vi "SDCCB Send Command.vi"(0 "VISA Ref":refnum<visa-resource-name>, 2 "Wait for Reply (T)":bool=TRUE, 7 "Command":string, 11 "Error In":errorcluster) -> (4 "VISA Ref Dup":refnum<visa-resource-name>, 8 "Reply":string, 15 "Error Out":errorcluster)   [LabVIEW 2020]
uses:
  <vilib>/Utility/error.llb/whitespace.ctl
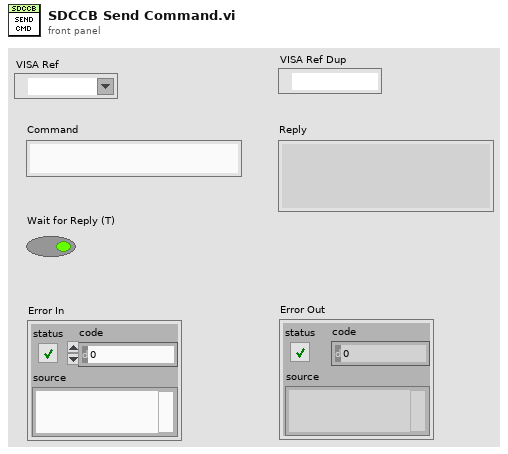
[diagram p1: front panel]
types:
  T1 = typedef "whitespace.ctl" = u16
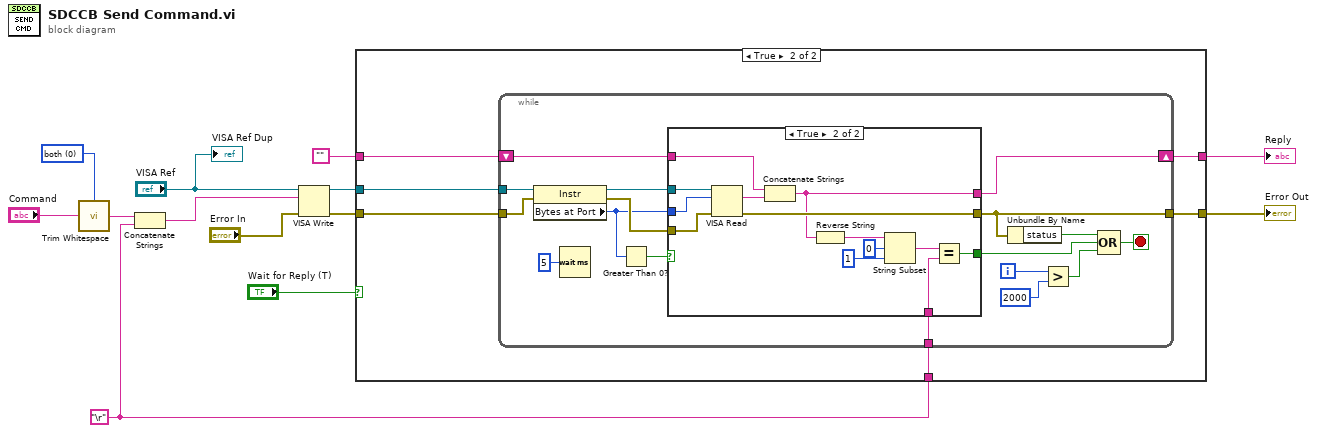
[diagram p0: block diagram]
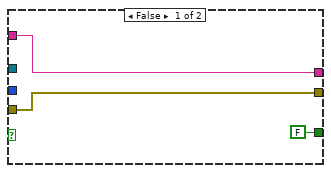
[diagram p3: hidden frame]
diagram:
  w1 = "\r"
  w12 = T1 0 items=["both", "start of string", "end of string"] ("location (both)")
  n1 = call <vilib>:"Trim Whitespace.vi"("string"="Command", "location (both)"=w12) -> ("trimmed string"=w11:string)
  n2 = Concatenate Strings(w11, w1) -> (w10:string)
  n3 = VISA Write(VISA resource name="VISA Ref", write buffer=w10, error in (no error)="Error In") -> (VISA resource name out=w9:refnum<visa-resource-name>, error out=w8:errorcluster)  [unwired: 1 out]
  n4 = case shown="True" "Wait for Reply (T)" {
    tunnel: w9 -> [_ w18]
    tunnel: w8 -> [w15 w17]
    tunnel: "" -> [w14 w21]
    tunnel: [w14 w20] -> w2
    tunnel: [w15 w19] -> w4
    tunnel: w1 -> [_ w16]
    frame False {
    }
    frame True {
      n5 = while {
        tunnel: w18 -> [w38]
        tunnel: w17 -> [w37]
        shift-right: [w26] -> w20
        shift-left: w21 -> [w27]
        tunnel: [w23] -> w19
        tunnel: w16 -> [w22]
        i -> [w36]
        stop <- w33 stop-if-true
        n6 = property class="Instr"(reference=w38, error in=w37) -> (reference out=w29:refnum<visa-resource-name>, error out=w30:errorcluster, "Bytes at Port"=w28:u32)
        n7 = Wait (ms)(milliseconds to wait=u32 5) -> ()  [unwired: 1 out]
        n8 = Greater Than 0?(x=w28) -> (x > 0?=w31:bool)
        n9 = case shown="True" w31 {
          tunnel: w30 -> [w40 w53]
          tunnel: w29 -> [_ w54]
          tunnel: w28 -> [_ w52]
          tunnel: w27 -> [w41 w51]
          tunnel: [w41 w48] -> w26
          tunnel: [w40 w49] -> w23
          tunnel: [FALSE w43] -> w24
          tunnel: w22 -> [_ w42]
          frame False {
          }
          frame True {
            n10 = VISA Read(VISA resource name=w54, byte count=w52, error in (no error)=w53) -> (read buffer=w50:string, error out=w49:errorcluster)  [unwired: 2 out]
            n11 = Concatenate Strings(w51, w50) -> (w48:string)
            n12 = Reverse String(1:w48) -> (0:w47:string)
            n13 = String Subset(string=w47, offset (0)=0, length (rest)=1 ("length (rest)")) -> (substring=w44:string)
            n14 = Equal?(x=w44, y=w42) -> (x = y?=w43:bool)
          }
        }
        n15 = Unbundle By Name(w23) -> ("status"=w25:bool)
        n16 = Greater?(x=w36, y=2000) -> (0:w34:bool)
        n17 = Compound Arithmetic op=OR(w25, w24, w34) -> (w33:bool)
      }
    }
  }
  "Reply" <- w2
  "Error Out" <- w4
  "VISA Ref Dup" <- "VISA Ref"
